vi "Field_Calc_Robot_Pixel_Location.vi"(4 "Y Conv":dbl, 6 "X Conv":dbl, 9 "Y  INCHES":dbl, 11 "X INCHES":dbl) -> (1 "Top Pixel":dbl, 3 "Left Pixel":dbl)   [LabVIEW 2019]
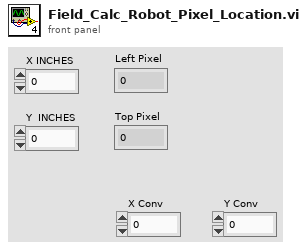
[diagram p1: front panel]
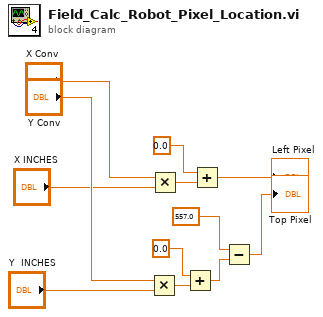
[diagram p0: block diagram]
diagram:
  n1 = Multiply(x="Y Conv", y="Y  INCHES") -> (x*y=w3:dbl)
  n2 = Multiply(x="X Conv", y="X INCHES") -> (x*y=w1:dbl)
  n3 = Add(x=0.0, y=w3) -> (x+y=w7:dbl)
  n4 = Add(x=0.0, y=w1) -> (x+y=→"Left Pixel":dbl)
  n5 = Subtract(x=557.0, y=w7) -> (x-y=→"Top Pixel":dbl)
